vi "LaneExtractor.vi"() -> ()   [LabVIEW 2024]
uses:
  <vilib>/userDefined/High Color/IMAQdx.ctl
  <vilib>/Python/Open Venv Python Session.vi
  <vilib>/vision/NI_Vision_Development_Module.lvlib
  <vilib>/vision/driver/NI_Vision_Acquisition_Software.lvlib
panel:
  in  "Session In":T1
  out "error out 2":errorcluster
  out "error out":errorcluster
  out "return value":string
  out "python_error":errorcluster
  out "Image":T2(plugin-control)
  in  "stop":bool
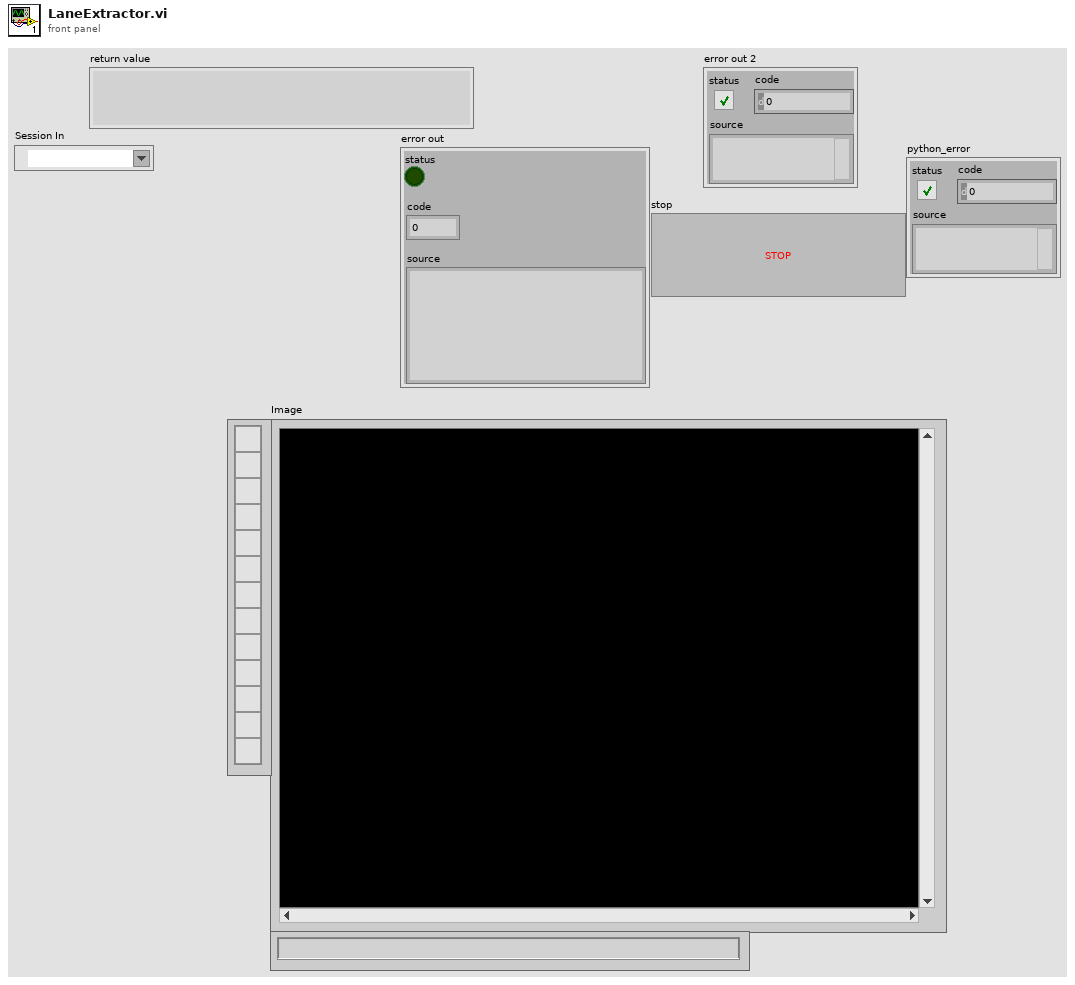
[diagram p1: front panel]
types:
  T1 = typedef "IMAQdx.ctl" = refnum<k21>
  T2 = typedef "IMAQ Image.ctl" = refnum<image>
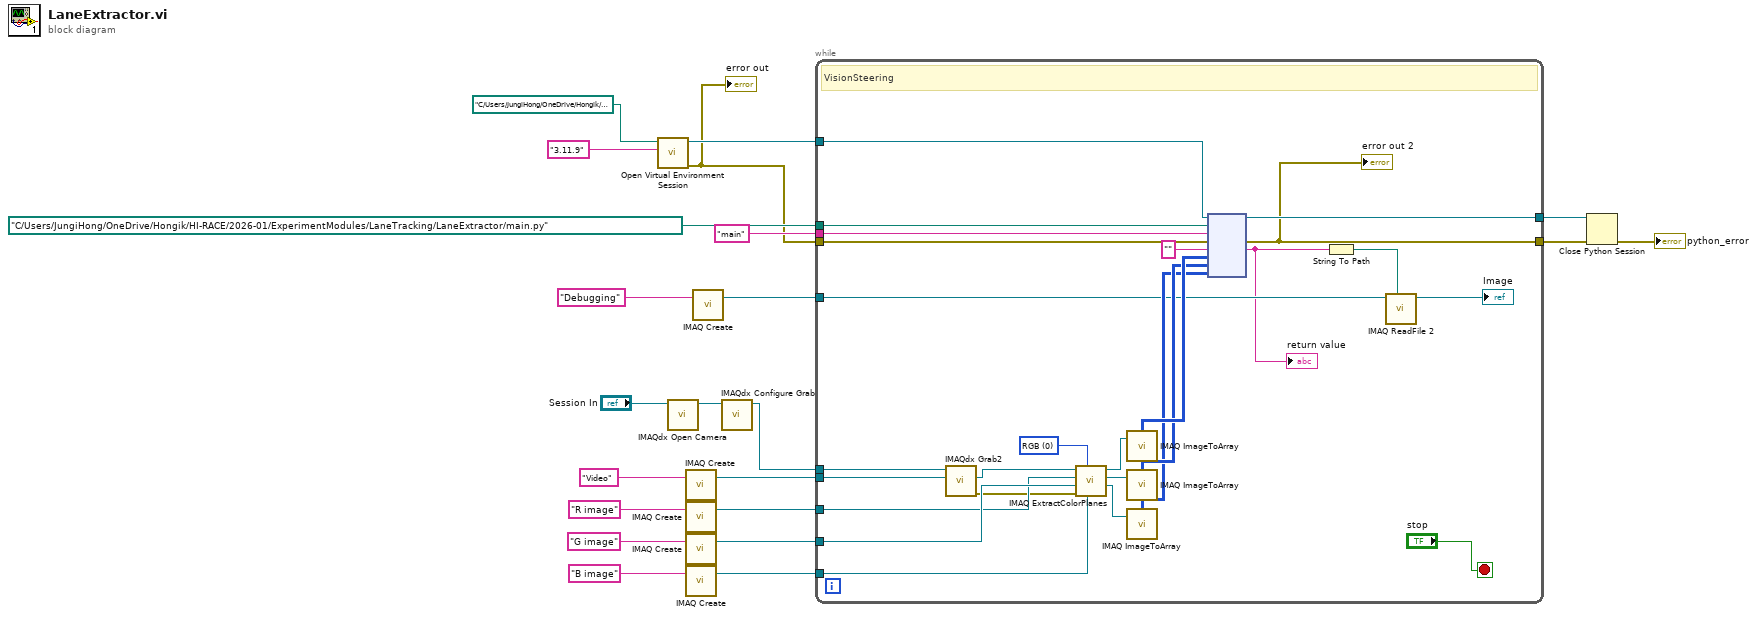
[diagram p0: block diagram]
diagram:
  n1 = call-poly <vilib>:"Open Virtual Environment Session.vi"("Python version"="3.11.9", "Env path"=path "C:/Users/JungiHong/OneDrive/Hongik/HI-RACE/2026-01/.venv") -> ("error out"=w4:errorcluster, "session out"=w20:refnum<k35>)  [unwired: 8 in]
  "error out" <- w4
  n2 = call <vilib>:"IMAQdx Open Camera.vi"("Session In"="Session In") -> ("Session Out"=w2:T1)  [unwired: 9 in, 1 out]
  n3 = call "IMAQ Create"("Image Name"="Video") -> ("New Image"=w21:T2)  [unwired: 4 in, 1 out]
  n4 = call "IMAQ Create"("Image Name"="R image") -> ("New Image"=w9:T2)  [unwired: 4 in, 1 out]
  n5 = call "IMAQ Create"("Image Name"="G image") -> ("New Image"=w10:T2)  [unwired: 4 in, 1 out]
  n6 = call "IMAQ Create"("Image Name"="B image") -> ("New Image"=w11:T2)  [unwired: 4 in, 1 out]
  n7 = call "IMAQ Create"("Image Name"="Debugging") -> ("New Image"=w15:T2)  [unwired: 4 in, 1 out]
  n8 = call <vilib>:"IMAQdx Configure Grab.vi"("Session In"=w2) -> ("Session Out"=w1:T1)  [unwired: 9 in, 1 out]
  n9 = while {
    tunnel: w21 -> [w25]
    tunnel: w20 -> [w47]
    tunnel: [w46] -> w17
    tunnel: w15 -> [w30]
    tunnel: w11 -> [w40]
    tunnel: w10 -> [w39]
    tunnel: w9 -> [w38]
    tunnel: path "C:/Users/JungiHong/OneDrive/Hongik/HI-RACE/2026-01/ExperimentModules/LaneTracking/LaneExtractor/main.py" ("module in") -> [w34]
    tunnel: "main" ("module out") -> [w33]
    tunnel: w4 -> [w32]
    tunnel: [w31] -> w6
    tunnel: w1 -> [w26]
    stop <- "stop" stop-if-true
    w41 = u16 0 items=["RGB", "HSL", "HSV", "HSI"] ("Color Mode")
    # "VisionSteering"
    n10 = call <vilib>:"IMAQdx Grab2.vi"("Image In"=w25, "Session In"=w26) -> ("error out"=w24:errorcluster, "Image Out"=w23:T2)  [unwired: 6 in, 2 out]
    n11 = call "IMAQ ExtractColorPlanes"("Blue or Luma or Val or Inten Plane"=w40, "Color Mode"=w41, "error in (no error)"=w24, "Green or Sat Plane"=w39, "Red or Hue Plane"=w38, "Image Src"=w23) -> ("Blue or Luma or Val or Inten Plane out"=w44:T2, "Green or Sat Plane out"=w43:T2, "Red or Hue Plane out"=w42:T2)  [unwired: 2 in, 1 out]
    n12 = call "IMAQ ImageToArray"("Image"=w42) -> ("Image Pixels (U8)"=w37:u8[][])  [unwired: 3 in, 4 out]
    n13 = call "IMAQ ImageToArray"("Image"=w43) -> ("Image Pixels (U8)"=w36:u8[][])  [unwired: 3 in, 4 out]
    n14 = call "IMAQ ImageToArray"("Image"=w44) -> ("Image Pixels (U8)"=w35:u8[][])  [unwired: 3 in, 4 out]
    n15 = node(w47, w34, w33, w32, "", w37, w36, w35) -> (w46:refnum<k35>, w31:errorcluster, w28:string)  [unwired: 3 in, 2 out]
    "return value" <- w28
    "error out 2" <- w31
    n16 = String To Path(string=w28) -> (path=w27:path)
    n17 = call "IMAQ ReadFile 2"("File Path"=w27, "Image"=w30) -> ("Image Out"=→"Image":T2)  [unwired: 5 in, 4 out]
  }
  n18 = Close Python Session(session in=w17, error in=w6) -> (11:→"python_error":errorcluster)
